vi "License Generator.vi"(8 "error in (no error)":errorcluster) -> (0 "error out":errorcluster)   [LabVIEW 2021]
uses:
  Controls/License Types.ctl
  Controls/License File Data.ctl
  Controls/License Generator States.ctl
panel:
  out "Sensor ID":string
  in  "License File Name":string="Customer"
  in  "Create License":bool
  in  "Choose License Type":T1=enum."Professional"
  in  "Evaluation Period":u16 max=365
  in  "Help":bool
  out "Requested Date":string
  out "Phone":string
  out "Email":string
  out "Computer ID":string
  out "Organization Name":string
  out "Name":string
  in  "License Request Form Path":path
  # "License Generator"
  # "License Form Data"
  # "Generate License"
  # "Days"
  # "Days"
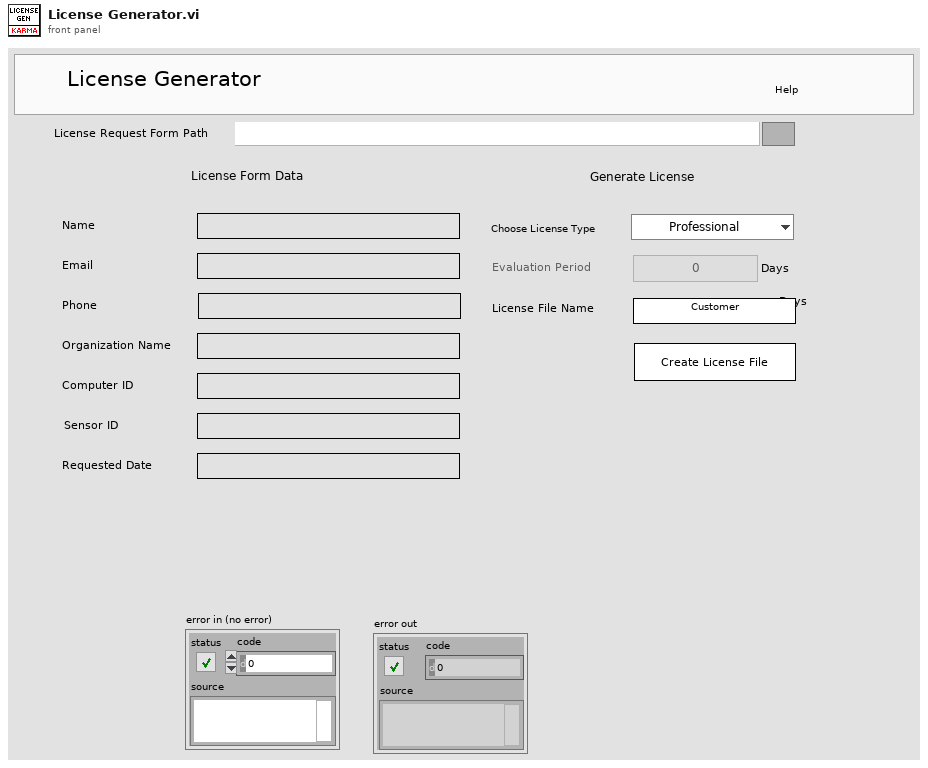
[diagram p1: front panel]
types:
  T1 = typedef "License Types.ctl" = enum16{"Evaluation", "Professional"}
  T2 = typedef "License File Data.ctl" = cluster{"Computer ID":string, "License Requested Date":string, "License Generated Date":string, "License Type":T1, "Evaluation Period":string, "License Generated Time":timestamp, "Sensor Serial Number":string}
  T3 = cluster{"License File Data":T2, "License Form Path":path}
  T4 = typedef "License Generator States.ctl" = enum16{"Poll", "Initialize", "Get Form Data", "Create License", "Error", "Exit"}
  T5 = enum8{"Enabled", "Disabled", "Disabled and Grayed Out"}
  T6 = typedef "License Request Form.ctl" = cluster{"Name":string, "Email":string, "Phone":string, "Computer ID":string, "Org Name":string, "Created Date":string, "Sensor ID":string}
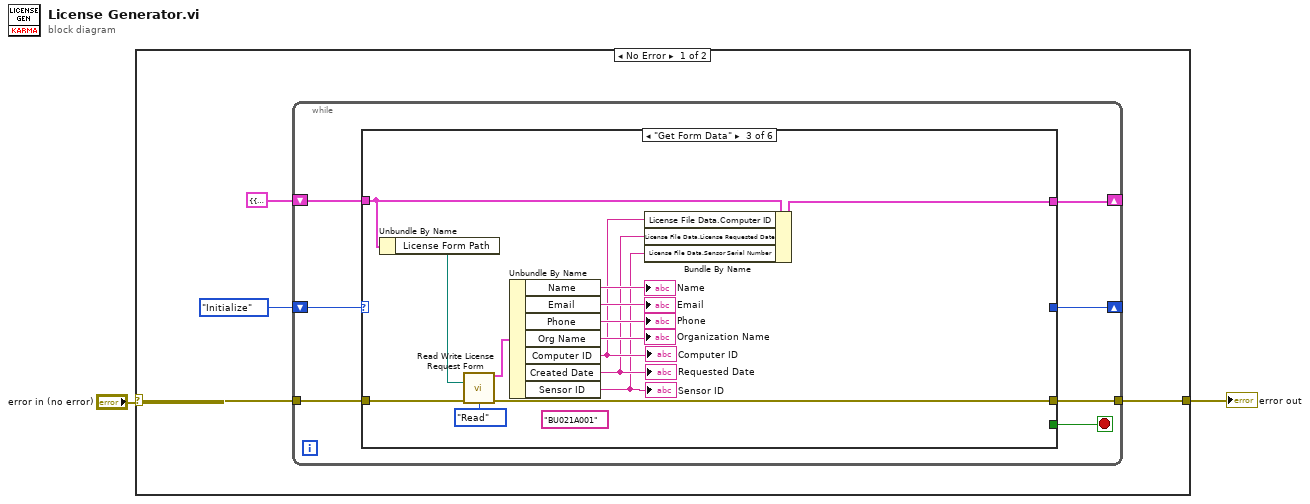
[diagram p0: block diagram]
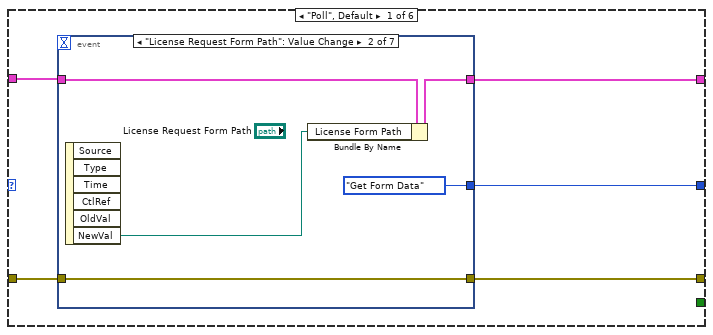
[diagram p2: hidden frame]
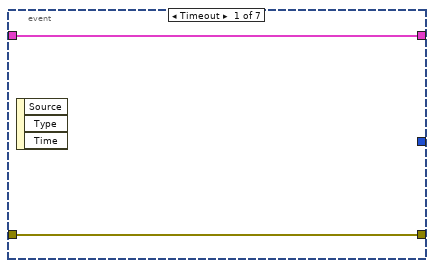
[diagram p3: hidden frame]
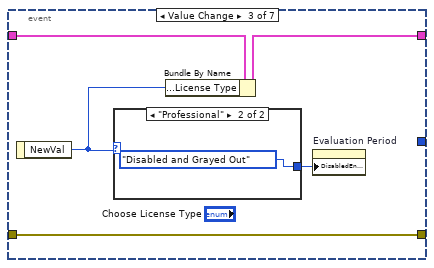
[diagram p4: hidden frame]
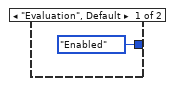
[diagram p5: hidden frame]
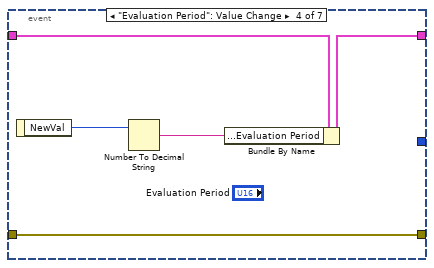
[diagram p6: hidden frame]
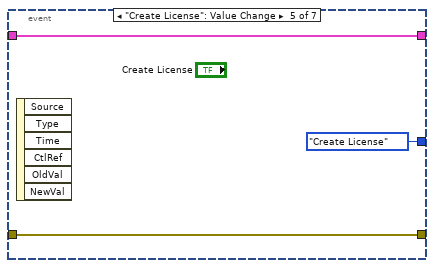
[diagram p7: hidden frame]
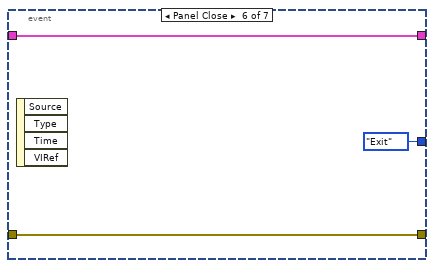
[diagram p8: hidden frame]
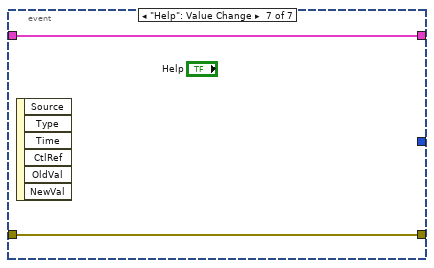
[diagram p9: hidden frame]
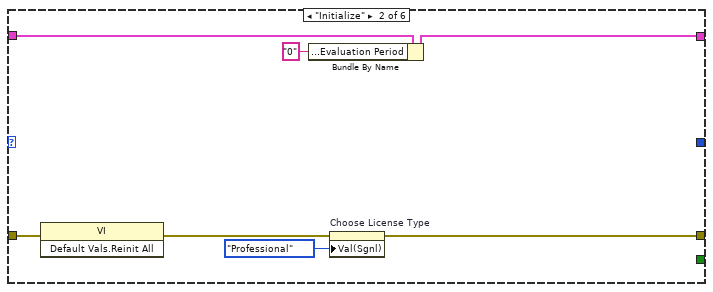
[diagram p10: hidden frame]
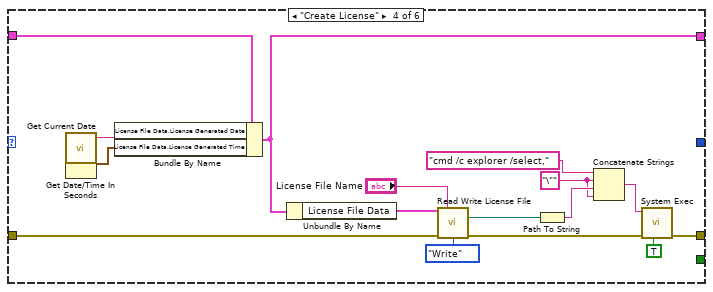
[diagram p11: hidden frame]
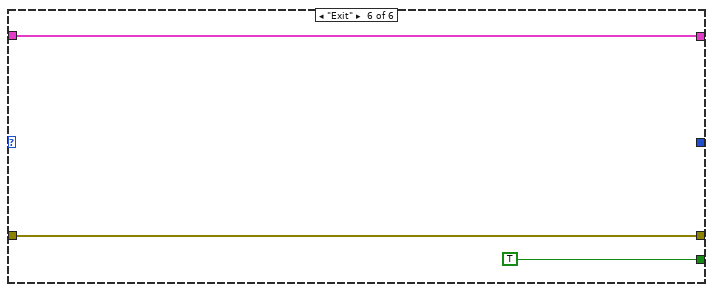
[diagram p13: hidden frame]
diagram:
  n1 = case shown="No Error" "error in (no error)" {
    selector: "error in (no error)" -> [w5 w88]
    tunnel: [w4 w88] -> w1
    frame No Error {
      n2 = while {
        shift-right: [w11] -> _
        shift-left: License_Generator_States."Initialize" -> [w13]
        tunnel: w5 -> [w10]
        tunnel: [w9] -> w4
        shift-right: [w7] -> _
        shift-left: T3 {"License File Data"={"Computer ID"="", "License Requested Date"="", "License Generated Date"="", "License Type"=enum."Evaluation", "Evaluation Period"="", "License Generated Time"=timestamp(0 s since 1904-01-01), "Sensor Serial Number"=""}, "License Form Path"=path ""} -> [w8]
        stop <- w12 stop-if-true
        n3 = case shown="\"Get Form Data\"" w13 {
          tunnel: [_ _ _ _ _ TRUE] -> w12
          tunnel: [w18 _ _ _ _ _] -> w11
          tunnel: w10 -> [w17 w52 w66 w79 w83 w85]
          tunnel: [w16 w46 w65 w69 w83 w85] -> w9
          tunnel: w8 -> [w15 w51 w55 w82 w84 w86]
          tunnel: [w14 w50 w58 w80 w84 w86] -> w7
          frame "Poll", Default {
            n4 = event shown="[1] \"License Request Form Path\": Value Change" {
              selector: _ -> [_ _ _ _ _ _ _]
              dyn-events: _ -> [_ _ _ _ _ _ _]
              timeout: _ -> [_ _ _ _ _ _ _]
              tunnel: [_ License_Generator_States."Get Form Data" _ _ License_Generator_States."Create License" License_Generator_States."Exit" _] -> w18
              tunnel: w17 -> [w20 w24 w30 w37 w40 w43 w45]
              tunnel: [w20 w24 w30 w37 w40 w43 w45] -> w16
              tunnel: w15 -> [w19 w23 w28 w36 w39 w41 w44]
              tunnel: [w19 w22 w27 w35 w39 w41 w44] -> w14
              event Timeout {
                n5 = event-data() -> ()  [unwired: 1 in, 3 out]
              }
              event "License Request Form Path": Value Change {
                n6 = event-data() -> ("NewVal"=w21:path)  [unwired: 1 in, 5 out]
                n7 = Bundle By Name(cluster=w23, "License Form Path"=w21) -> (w22:T3)
              }
              event Value Change {
                n8 = event-data() -> ("NewVal"=w26:T1)  [unwired: 1 in]
                n9 = case shown="\"Professional\"" w26 {
                  tunnel: [T5."Enabled" ("Disabled") T5."Disabled and Grayed Out" ("Disabled")] -> w29
                  frame "Evaluation", Default {
                  }
                  frame "Professional" {
                  }
                }
                n10 = Bundle By Name(cluster=w28, "License File Data.License Type"=w26) -> (w27:T3)
                n11 = property on="Evaluation Period" class="DigNum (strict)"("DisabledEnum"=w29) -> ()  [unwired: 2 in, 2 out]
              }
              event "Evaluation Period": Value Change {
                n12 = event-data() -> ("NewVal"=w34:u16)  [unwired: 1 in]
                n13 = Number To Decimal String(number=w34) -> (decimal integer string=w33:string)  [unwired: 1 in]
                n14 = Bundle By Name(cluster=w36, "License File Data.Evaluation Period"=w33) -> (w35:T3)
              }
              event "Create License": Value Change {
                n15 = event-data() -> ()  [unwired: 1 in, 6 out]
              }
              event Panel Close {
                n16 = event-data() -> ()  [unwired: 1 in, 4 out]
              }
              event "Help": Value Change {
                n17 = event-data() -> ()  [unwired: 1 in, 6 out]
              }
            }
          }
          frame "Initialize" {
            n18 = invoke class="VI" method="Default Vals.Reinit All"(error in=w52) -> (error out=w48:errorcluster)  [unwired: 2 in, 2 out]
            n19 = Bundle By Name(cluster=w51, "License File Data.Evaluation Period"="0") -> (w50:T3)
            n20 = property on="Choose License Type" class="Enum (strict)"(error in=w48, "Val(Sgnl)"=License_Types."Professional" ("Value (Signaling)")) -> (error out=w46:errorcluster)  [unwired: 1 in, 1 out]
          }
          frame "Get Form Data" {
            (unwired) "BU021A001" ("Sensor ID")
            n21 = Unbundle By Name(w55) -> ("License Form Path"=w54:path)
            n22 = call "Read Write License Request Form.vi"("Info File Path"=w54, "Error in (no error)"=w66, "Operation"=enum16{"Write", "Read"}."Read") -> ("License Form Out"=w63:T6, "Error out"=w65:errorcluster)  [unwired: 10 in, 1 out]
            n23 = Unbundle By Name(w63) -> ("Name"=→"Name":string, "Email"=→"Email":string, "Phone"=→"Phone":string, "Org Name"=→"Organization Name":string, "Computer ID"=w57:string, "Created Date"=w56:string, "Sensor ID"=w53:string)
            "Computer ID" <- w57
            "Requested Date" <- w56
            "Sensor ID" <- w53
            n24 = Bundle By Name(cluster=w55, "License File Data.Computer ID"=w57, "License File Data.License Requested Date"=w56, "License File Data.Sensor Serial Number"=w53) -> (w58:T3)
          }
          frame "Create License" {
            w74 = "\"" ("string")
            n25 = call "Get Current Date.vi"() -> ("Date String"=w81:string)  [unwired: 8 in]
            n26 = Get Date/Time In Seconds() -> (seconds since 1Jan1904=w67:timestamp)
            n27 = Bundle By Name(cluster=w82, "License File Data.License Generated Date"=w81, "License File Data.License Generated Time"=w67) -> (w80:T3)
            n28 = Unbundle By Name(w80) -> ("License File Data"=w78:T2)
            n29 = call "Read Write License File.vi"("License File Data"=w78, "License File Name"="License File Name", "Error in (no error)"=w79, "Operation"=enum16{"Write", "Read"}."Write") -> ("License File Path"=w68:path, "Error out"=w70:errorcluster)  [unwired: 9 in, 1 out]
            n30 = Path To String(path=w68) -> (string=w75:string)
            n31 = Concatenate Strings("cmd /c explorer /select," ("string"), w74, w75, w74) -> (w71:string)
            n32 = call <vilib>:"System Exec.vi"("run minimized? (F)"=TRUE, "error in (no error)"=w70, "command line"=w71) -> ("error out"=w69:errorcluster)  [unwired: 5 in, 3 out]
          }
          frame "Error" {
          }
          frame "Exit" {
          }
        }
      }
    }
    frame Error {
    }
  }
  "error out" <- w1
